vi "Wash State For Command.vi"(11 "Command":T2) -> (3 "Queue Data for Command":T1)   [LabVIEW 2018]
uses:
  Command.ctl
  MessageQueueData.ctl
  WashState.ctl
  Position.ctl
panel:
  in  "data":T1
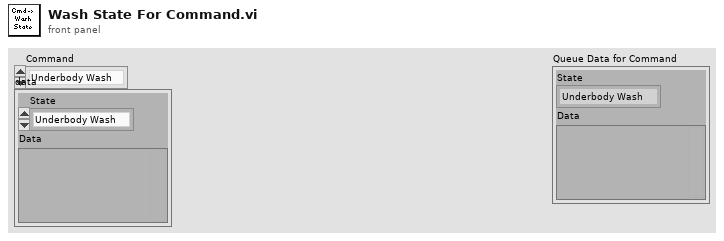
[diagram p1: front panel]
types:
  T1 = typedef "MessageQueueData.ctl" = cluster{"State":T2, "Data":variant}
  T2 = typedef "Command.ctl" = enum16{"Underbody Wash", "Soap Application", "Main High-Pressure Wash", "Clear Water Rinse", "Air Dry Cycle", "Stop"}
  T3 = typedef "WashState.ctl" = cluster{"Time Remaining":i32, "LastTickCount":i32, "Required Vehicle Position":T4}
  T4 = typedef "Position.ctl" = enum32{"Under Body Wash Position", "Main Wash Position", "Air Dry Position"}
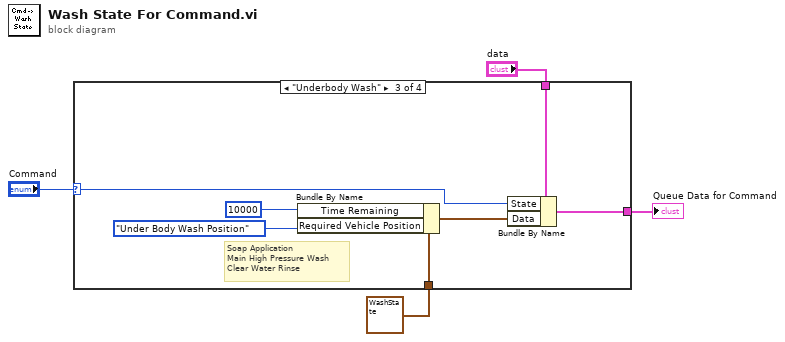
[diagram p0: block diagram]
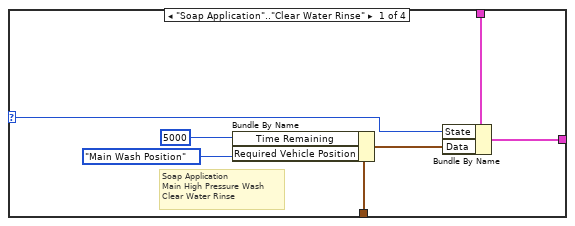
[diagram p2: hidden frame]
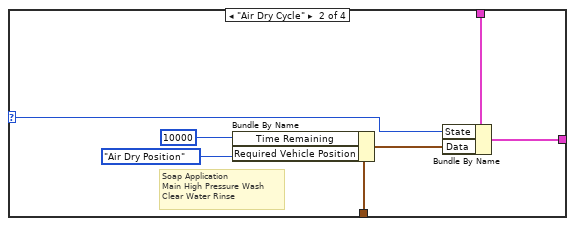
[diagram p3: hidden frame]
diagram:
  n1 = case shown="\"Underbody Wash\"" "Command" {
    selector: "Command" -> [w7 w14 w21 _]
    tunnel: T3 {"Time Remaining"=0, "LastTickCount"=-1, "Required Vehicle Position"=enum."Under Body Wash Position"} ("WashState") -> [w9 w16 w23 _]
    tunnel: [w6 w13 w20 _] -> w1
    tunnel: "data" -> [w5 w12 w19 _]
    frame "Soap Application".."Clear Water Rinse" {
      # "Soap Application\nMain High Pressure Wash\nClear Water Rinse"
      n2 = Bundle By Name(cluster=w9, "Time Remaining"=5000, "Required Vehicle Position"=Position."Main Wash Position" ("Vehicle Position")) -> (w8:T3)
      n3 = Bundle By Name(cluster=w5, "State"=w7, "Data"=w8) -> (w6:T1)
    }
    frame "Air Dry Cycle" {
      # "Soap Application\nMain High Pressure Wash\nClear Water Rinse"
      n4 = Bundle By Name(cluster=w16, "Time Remaining"=10000, "Required Vehicle Position"=Position."Air Dry Position" ("Vehicle Position")) -> (w15:T3)
      n5 = Bundle By Name(cluster=w12, "State"=w14, "Data"=w15) -> (w13:T1)
    }
    frame "Underbody Wash" {
      # "Soap Application\nMain High Pressure Wash\nClear Water Rinse"
      n6 = Bundle By Name(cluster=w23, "Time Remaining"=10000, "Required Vehicle Position"=Position."Under Body Wash Position" ("Vehicle Position")) -> (w22:T3)
      n7 = Bundle By Name(cluster=w19, "State"=w21, "Data"=w22) -> (w20:T1)
    }
    frame "Stop" {
    }
  }
  "Queue Data for Command" <- w1
